vi "MasterVI.vi"() -> ()   [LabVIEW 2017]
panel:
  in  "Offset (V)":dbl
  in  "Total Y-axis Distance (mm)":dbl
  in  "File Save Path":string="C:\\Users\\Carlos\\Documents\\Garcia_Carlos"
  in  "Y Axis Calibration Constant":dbl
  in  "Distance/Sample (mm)":dbl
  in  "Axis# 2":i16 min=0 max=2 step=1
  in  "Forward/Reverse":bool
  in  "X Axis Calibration Constant":dbl
  in  "Total X Dist (mm)":dbl
  out "5V Indicator":bool
  in  "Axis#":i16 min=0 max=2 step=1
  in  "Forward/Reverse":bool
  in  "Initial Flow Diameter (mm)":dbl
  # "Y Axis Settings"
  # "X Axis Settings"
  # "Save File Location"
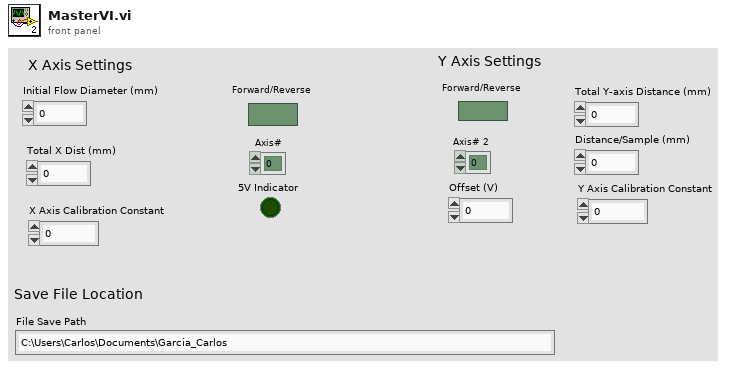
[diagram p1: front panel]
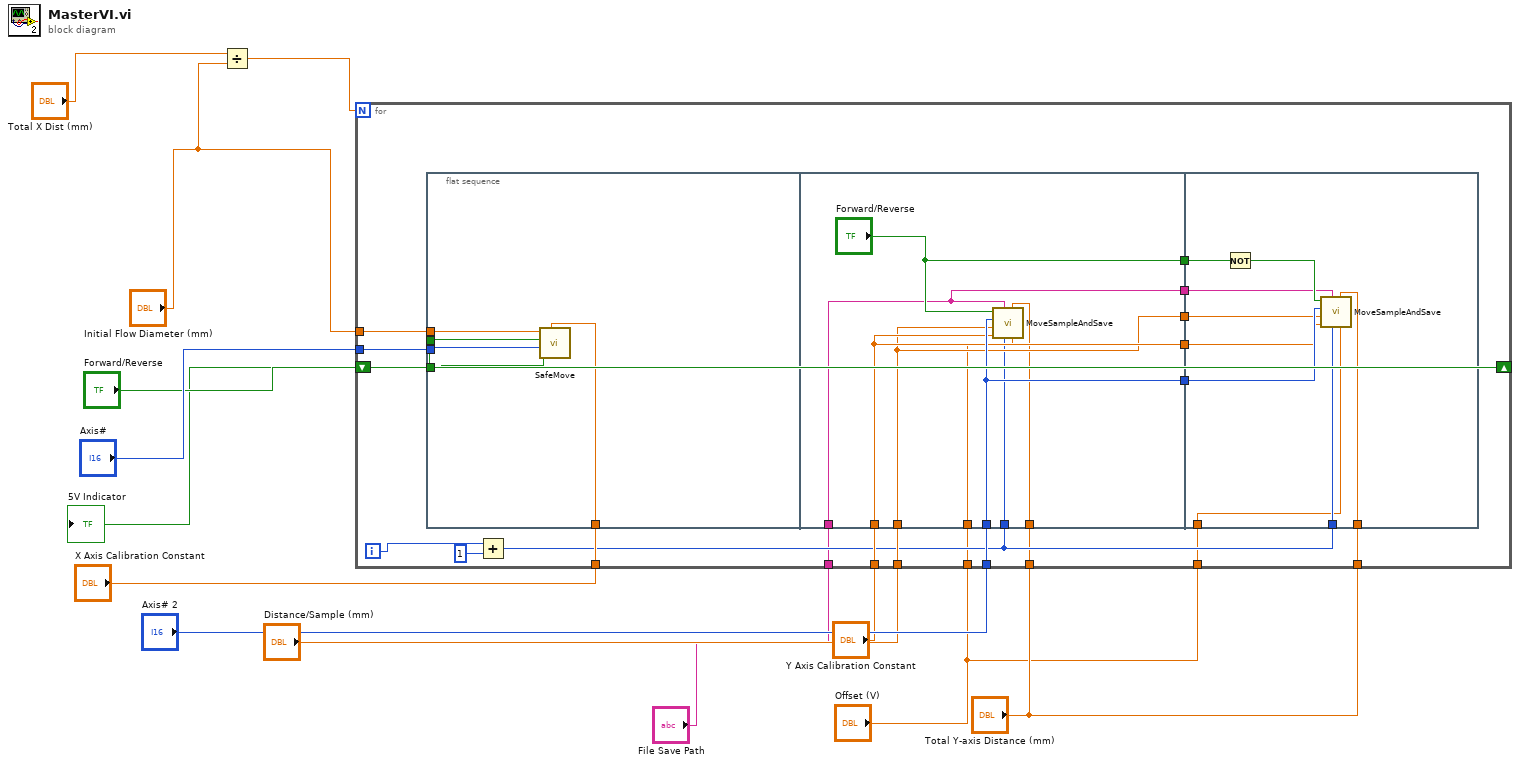
[diagram p0: block diagram]
diagram:
  n1 = Divide(x="Total X Dist (mm)", y="Initial Flow Diameter (mm)") -> (x/y=w6:dbl)
  n2 = for {
    N: w6 -> [_]
    tunnel: "Axis#" -> [w30]
    tunnel: "Initial Flow Diameter (mm)" -> [w27]
    tunnel: "X Axis Calibration Constant" -> [w26]
    tunnel: "Axis# 2" -> [w25]
    tunnel: "Distance/Sample (mm)" -> [w24]
    tunnel: "Y Axis Calibration Constant" -> [w23]
    shift-right: [w28] -> w11
    shift-left: "Forward/Reverse" -> [w29]
    tunnel: "File Save Path" -> [w19]
    tunnel: "Total Y-axis Distance (mm)" -> [w17]
    tunnel: "Total Y-axis Distance (mm)" -> [w16]
    tunnel: "Offset (V)" -> [w15]
    tunnel: "Offset (V)" -> [w14]
    i -> [w22]
    n3 = flat-sequence {
      tunnel: w30 -> [w37]
      tunnel: w29 -> [w38]
      tunnel: [w36] -> w28
      tunnel: w27 -> [w39]
      tunnel: w26 -> [w35]
      tunnel: ["Forward/Reverse"] -> w34
      tunnel: w25 -> [w46]
      tunnel: [w46] -> w33
      tunnel: w24 -> [w44]
      tunnel: [w45] -> w32
      tunnel: w23 -> [w45]
      tunnel: [w44] -> w31
      tunnel: w20 -> [w43]
      tunnel: w19 -> [w42]
      tunnel: [w42] -> w18
      tunnel: w17 -> [w41]
      tunnel: w15 -> [w40]
      tunnel: w34 -> [w56]
      tunnel: w33 -> [w54]
      tunnel: w32 -> [w53]
      tunnel: w31 -> [w52]
      tunnel: w20 -> [w51]
      tunnel: w18 -> [w50]
      tunnel: w16 -> [w49]
      tunnel: w14 -> [w48]
      frame #0 {
        n4 = call "SafeMove.vi"("Calibration Constant"=w35, "Axis#"=w37, "Forward/Reverse"=w38, "Total Distance (mm)"=w39) -> ("5V Indicator"=w36:bool)  [unwired: 7 in]
      }
      frame #1 {
        n5 = call "MoveSampleAndSave.vi"("Offset (V)"=w40, "Total Y-axis Distance (mm)"=w41, "x (in units of D)"=w43, "File Save Path"=w42, "Y Calibration Constant"=w45, "Y-axis Distance/Sample"=w44, "Axis#"=w46, "Forward/Reverse"="Forward/Reverse") -> ()  [unwired: 4 in]
      }
      frame #2 {
        n6 = Not(x=w56) -> (.not. x?=w55:bool)
        n7 = call "MoveSampleAndSave.vi"("Offset (V)"=w48, "Total Y-axis Distance (mm)"=w49, "x (in units of D)"=w51, "File Save Path"=w50, "Y Calibration Constant"=w53, "Y-axis Distance/Sample"=w52, "Axis#"=w54, "Forward/Reverse"=w55) -> ()  [unwired: 4 in]
      }
    }
    n8 = Add(x=w22, y=1) -> (x+y=w20:i32)
  }
  "5V Indicator" <- w11
